vi "Periodic Tasks.vi"() -> ()   [LabVIEW 2011]
doc: "This VI runs in parallel to other tasks. It can contain as many user-defined periodic loops as you need. These can carry out PID or other sorts of timed response."
uses:
  <vilib>/Rock Robotics/SystemInterfaces/Utilities/FPGA_UtilitiesLED State.ctl
  <vilib>/Rock Robotics/SystemInterfaces/Utilities/FPGA_UtilitiesLED Source.ctl
  Robot Global Data.vi
  <vilib>/Rock Robotics/WPI/Relay/WPI_RelayValue.ctl
panel:
  in  "Reset Ball":bool
  in  "Home Speed":dbl=0.4
  out "Auton Recording":bool
  in  "Turn on Record":bool
  in  "Auton Array":dbl[][](array[numeric])
  out "Ramp ACT Pot":dbl
  out "Right Rate":dbl
  out "Right Direction":bool
  out "Right Distance":dbl
  out "Shooter Encoder Distance":dbl
  out "Shooter Direction":bool
  out "Shooter Encoder Rate":dbl
  out "Left Rate":dbl
  out "Gyro Rate":dbl
  out "Gyro Angle":dbl
  out "Left Direction":bool
  out "Left Distance":dbl
  # "Auton Recording"
  # "Sensor Feedback"
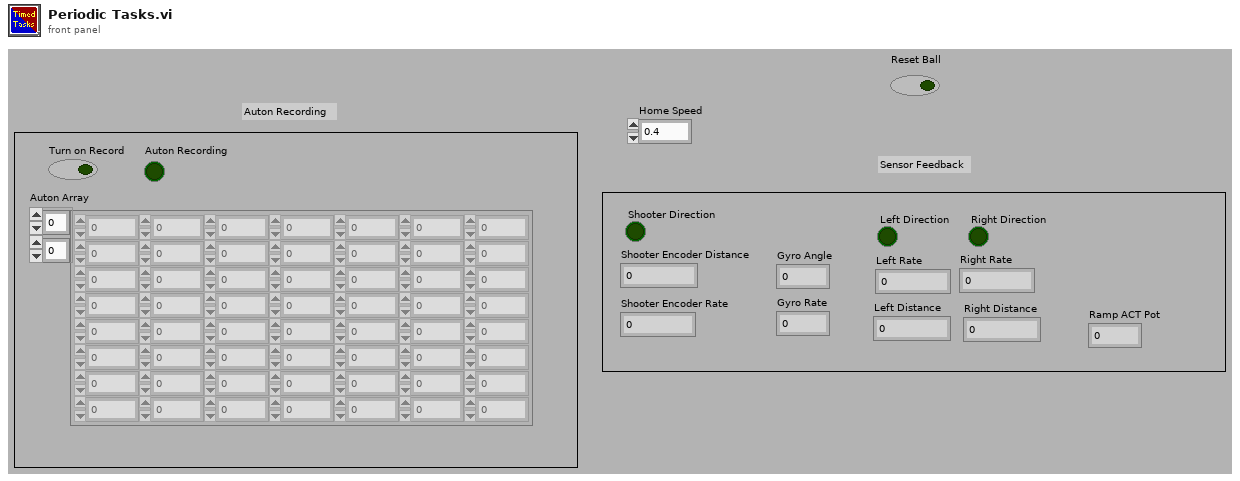
[diagram p1: front panel]
types:
  T1 = typedef "WPI_RelayValue.ctl" = enum16{"Off", "On", "Forward", "Reverse"}
  T2 = typedef "WPI_AnalogChannelDevRef.ctl" = cluster{"DevStatus":errorcluster, "Analog Module":T3, "Analog Channel":T4}
  T3 = typedef "FPGA_TypedefAnalogModule.ctl" = enum16{"Analog Module 1", "Analog Module 2"}
  T4 = typedef "FPGA_AIChannel.ctl" = enum8{"AI 1", "AI 2", "AI 3", "AI 4", "AI 5", "AI 6", "AI 7", "AI 8", "Invalid"}
  T5 = typedef "WPI_EncoderDevRef.ctl" = cluster{"DevStatus":errorcluster, "EncoderIndex":T6, "CounterIndex":T7, "DistancePerCount":dbl, "Decoding Type":T8}
  T6 = typedef "FPGA_EncoderIdx.ctl" = enum8{"Enc 0", "Enc 1", "Enc 2", "Enc 3", "Invalid"}
  T7 = typedef "FPGA_CounterCtrSystemIndex.ctl" = enum8{"Ctr 0", "Ctr 1", "Ctr 2", "Ctr 3", "Ctr 4", "Ctr 5", "Ctr 6", "Ctr 7", "Invalid"}
  T8 = typedef "WPI_EncoderType.ctl" = enum16{"1x", "2x", "4x"}
  T9 = typedef "WPI_GyroDevRef.ctl" = cluster{"DevStatus":errorcluster, "Analog Module":T3, "Analog Channel":T4, "Offset":dbl, "Gain (VoltsPerDegree/Second)":dbl}
  T10 = typedef "WPI_RelayDevRef.ctl" = cluster{"DevStatus":errorcluster, "Relay Channel":T11, "Digital Module":T12, "Relay Direction":T13}
  T11 = typedef "FPGA_DIORelayChannel.ctl" = enum8{"Relay 1", "Relay 2", "Relay 3", "Relay 4", "Relay 5", "Relay 6", "Relay 7", "Relay 8", "Invalid"}
  T12 = typedef "FPGA_TypedefDigitalModule.ctl" = enum16{"Digital Module 1", "Digital Module 2"}
  T13 = typedef "WPI_RelayDirection.ctl" = enum16{"Both directions", "Forward only", "Reverse only"}
  T14 = typedef "FPGA_UtilitiesLED State.ctl" = enum16{"Off", "On", "Toggle"}
  T15 = typedef "FPGA_UtilitiesLED Source.ctl" = enum16{"User LED", "FPGA LED"}
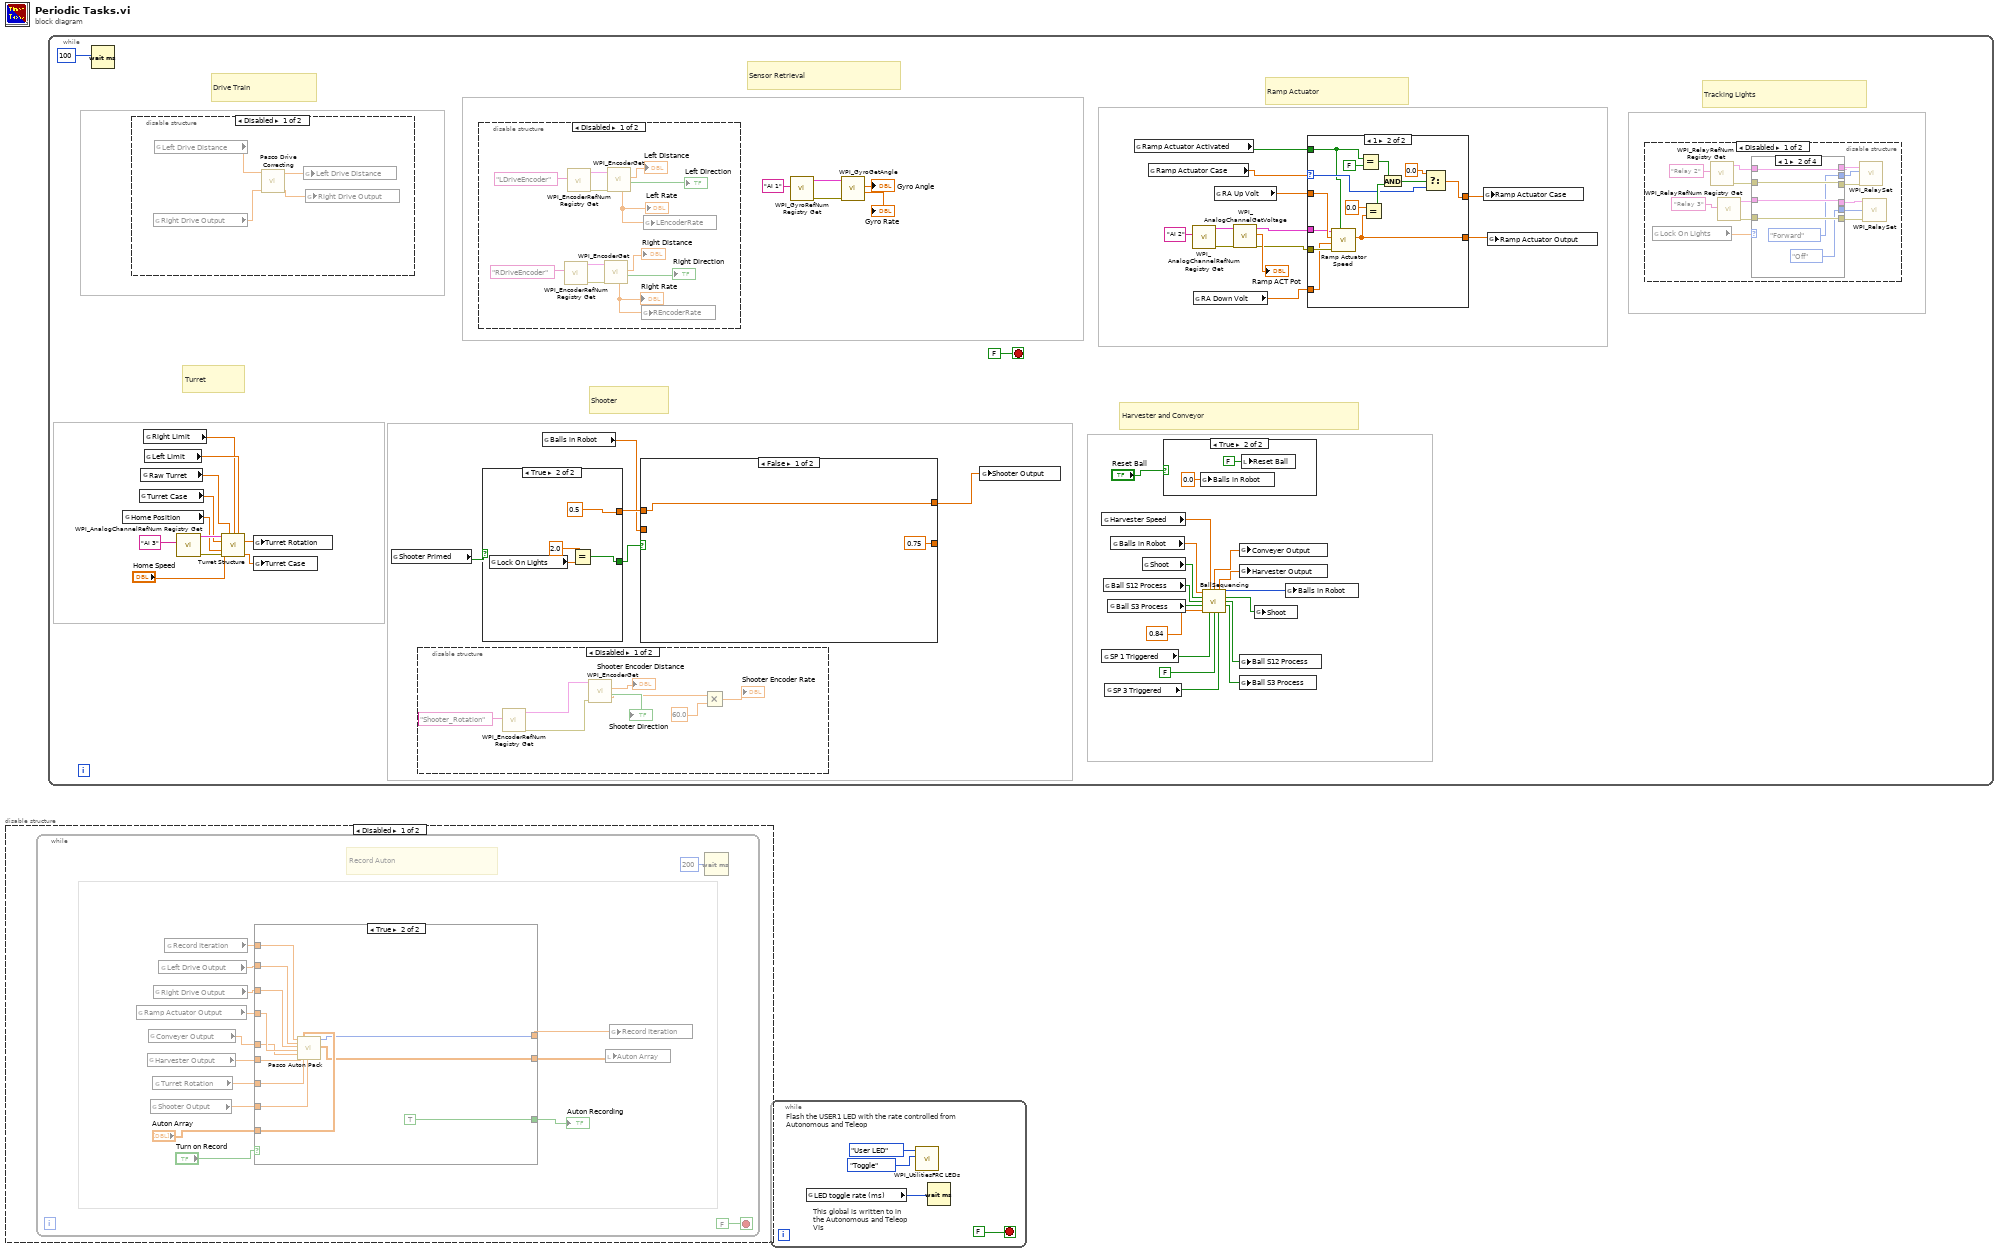
[diagram p0: block diagram]
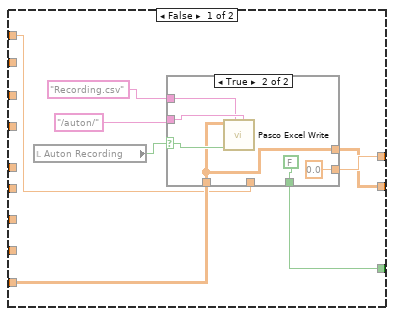
[diagram p2: hidden frame]
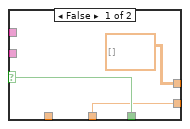
[diagram p3: hidden frame]
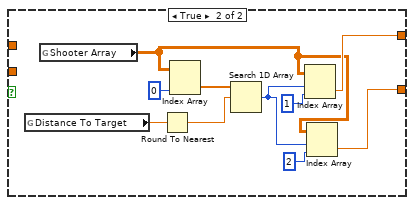
[diagram p5: hidden frame]
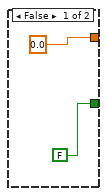
[diagram p6: hidden frame]
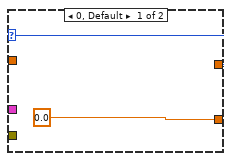
[diagram p8: hidden frame]
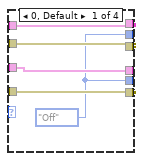
[diagram p10: hidden frame]
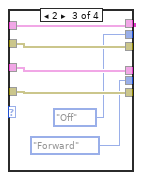
[diagram p11: hidden frame]
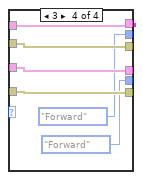
[diagram p12: hidden frame]
diagram:
  n1 = disable-structure shown="Disabled" {
    frame Disabled {
      n2 = while {
        stop <- FALSE stop-if-true
        # "Record Auton"
        n3 = global read "Robot Global Data.vi" "Ramp Actuator Output"() -> (w5:dbl)
        n4 = global read "Robot Global Data.vi" "Harvester Output"() -> (w7:dbl)
        n5 = global read "Robot Global Data.vi" "Conveyer Output"() -> (w6:dbl)
        n6 = global read "Robot Global Data.vi" "Shooter Output"() -> (w9:dbl)
        n7 = global read "Robot Global Data.vi" "Turret Rotation"() -> (w8:dbl)
        n8 = global read "Robot Global Data.vi" "Right Drive Output"() -> (w4:dbl)
        n9 = global read "Robot Global Data.vi" "Left Drive Output"() -> (w3:dbl)
        n10 = global read "Robot Global Data.vi" "Record Iteration"() -> (w2:dbl)
        n11 = case shown="True" "Turn on Record" {
          tunnel: w2 -> [w19 w44]
          tunnel: w3 -> [_ w43]
          tunnel: w4 -> [_ w42]
          tunnel: w5 -> [_ w41]
          tunnel: w6 -> [_ w40]
          tunnel: w7 -> [_ w39]
          tunnel: w8 -> [_ w38]
          tunnel: w9 -> [_ w37]
          tunnel: "Auton Array" -> [w20 w36]
          tunnel: [w16 w35] -> w12
          tunnel: [w17 w34] -> w13
          tunnel: [w18 TRUE] -> w14
          frame False {
            n12 = local read "Auton Recording"() -> (w21:bool)
            n13 = case shown="True" w21 {
              selector: w21 -> [w26 w31]
              tunnel: [w26 FALSE] -> w18
              tunnel: "/auton/" ("File Name") -> [_ w30]
              tunnel: "Recording.csv" ("Folder Location") -> [_ w29]
              tunnel: [w25 0.0 ("Record Iteration")] -> w17
              tunnel: w19 -> [w25 _]
              tunnel: w20 -> [_ w27]
              tunnel: [dbl[][] [] ("Auton Array") w27] -> w16
              frame False {
              }
              frame True {
                n14 = call "Pasco Excel Write.vi"("Folder Location"=w30, "File Name"=w29, "WriteToExcel"=w31, "2D data"=w27) -> ()  [unwired: 7 in, 1 out]
              }
            }
          }
          frame True {
            n15 = call "Pasco Auton Pack.vi"("Iterations"=w44, "Left Drive"=w43, "Right Drive"=w42, "RAMP ACT"=w41, "Conveyor"=w40, "Harvestor"=w39, "Auton Array"=w36, "Turret"=w38, "Shooter"=w37) -> ("Iteration Output"=w34:i32, "output array"=w35:dbl[][])  [unwired: 9 in]
          }
        }
        "Auton Recording" <- w14
        n16 = local write "Auton Array"(w12) -> ()
        n17 = global write "Robot Global Data.vi" "Record Iteration"(w13) -> ()
        n18 = Wait (ms)(milliseconds to wait=u32 200) -> ()  [unwired: 1 out]
      }
    }
    frame Enabled {
    }
  }
  n19 = while {
    stop <- FALSE stop-if-true
    # "Tracking Lights"
    # "Harvester and Conveyor"
    # "Shooter"
    # "Sensor Retrieval"
    # "Turret"
    # "Drive Train"
    # "Ramp Actuator"
    n20 = Wait (ms)(milliseconds to wait=u32 100) -> ()  [unwired: 1 out]
    n21 = global read "Robot Global Data.vi" "Home Position"() -> (w89:dbl)
    n22 = disable-structure shown="Disabled" {
      frame Disabled {
        n23 = global read "Robot Global Data.vi" "Right Drive Output"() -> (w182:dbl)
        n24 = global read "Robot Global Data.vi" "Left Drive Distance"() -> (w183:dbl)
        n25 = call "Pasco Drive Correcting.vi"("RightDriveOutput"=w182, "LeftDriveOutput"=w183) -> ("RightDriveOutput"=w180:dbl, "LeftDriveOutput"=w181:dbl)  [unwired: 8 in]
        n26 = global write "Robot Global Data.vi" "Left Drive Distance"(w181) -> ()
        n27 = global write "Robot Global Data.vi" "Right Drive Output"(w180) -> ()
      }
      frame Enabled {
      }
    }
    n28 = global read "Robot Global Data.vi" "Turret Case"() -> (w90:dbl)
    n29 = global read "Robot Global Data.vi" "Raw Turret"() -> (w88:dbl)
    n30 = global read "Robot Global Data.vi" "Right Limit"() -> (w71:dbl)
    n31 = global read "Robot Global Data.vi" "Left Limit"() -> (w72:dbl)
    n32 = call <vilib>:"WPI_AnalogChannelRefNum Registry Get.vi"("refnum name"="AI 3") -> ("error out"=w91:errorcluster, "AIDeviceRef"=w92:T2)  [unwired: 9 in]
    n33 = call "Turret Structure.vi"("AIDeviceRef"=w92, "Raw Turret"=w88, "upper limit"=w71, "lower limit"=w72, "Turret Case"=w90, "Home Speed"="Home Speed", "Home postion"=w89, "error in (no error)"=w91) -> ("Turret Output"=w87:dbl, "Turret Case Output"=w86:dbl)  [unwired: 6 in]
    n34 = global write "Robot Global Data.vi" "Turret Rotation"(w87) -> ()
    n35 = global write "Robot Global Data.vi" "Turret Case"(w86) -> ()
    n36 = global read "Robot Global Data.vi" "Shooter Primed"() -> (w58:bool)
    n37 = disable-structure shown="Disabled" {
      frame Disabled {
        n38 = call <vilib>:"WPI_EncoderRefNum Registry Get.vi"("refnum name"="Shooter_Rotation") -> ("error out"=w184:errorcluster, "EncoderDevRef"=w185:T5)  [unwired: 9 in]
        n39 = call <vilib>:"WPI_EncoderGet.vi"("error in (no error)"=w184, "EncoderDevRef"=w185) -> ("Direction"=→"Shooter Direction":bool, "Distance"=→"Shooter Encoder Distance":dbl, "Rate"=w188:dbl)  [unwired: 4 in, 3 out]
        n40 = Multiply(x=w188, y=60.0) -> (x*y=→"Shooter Encoder Rate":dbl)
      }
      frame Enabled {
      }
    }
    n41 = disable-structure shown="Disabled" {
      frame Disabled {
        n42 = call <vilib>:"WPI_EncoderRefNum Registry Get.vi"("refnum name"="RDriveEncoder") -> ("error out"=w136:errorcluster, "EncoderDevRef"=w135:T5)  [unwired: 9 in]
        n43 = call <vilib>:"WPI_EncoderRefNum Registry Get.vi"("refnum name"="LDriveEncoder") -> ("error out"=w142:errorcluster, "EncoderDevRef"=w141:T5)  [unwired: 9 in]
        n44 = call <vilib>:"WPI_EncoderGet.vi"("error in (no error)"=w136, "EncoderDevRef"=w135) -> ("Direction"=→"Right Direction":bool, "Distance"=→"Right Distance":dbl, "Rate"=w132:dbl)  [unwired: 4 in, 3 out]
        "Right Rate" <- w132
        n45 = call <vilib>:"WPI_EncoderGet.vi"("error in (no error)"=w142, "EncoderDevRef"=w141) -> ("Direction"=→"Left Direction":bool, "Distance"=→"Left Distance":dbl, "Rate"=w138:dbl)  [unwired: 4 in, 3 out]
        "Left Rate" <- w138
        n46 = global write "Robot Global Data.vi" "REncoderRate"(w132) -> ()
        n47 = global write "Robot Global Data.vi" "LEncoderRate"(w138) -> ()
      }
      frame Enabled {
      }
    }
    n48 = case shown="True" w58 {
      tunnel: [FALSE ("Shooter Primed") w110] -> w57
      tunnel: [0.0 0.5] -> w55
      frame False {
      }
      frame True {
        n49 = global read "Robot Global Data.vi" "Lock On Lights"() -> (w112:dbl)
        n50 = Equal?(x=2.0, y=w112) -> (x = y?=w110:bool)
      }
    }
    n51 = global read "Robot Global Data.vi" "Balls in Robot"() -> (w54:dbl)
    n52 = case shown="False" w57 {
      tunnel: [w97 w107] -> w56
      tunnel: w55 -> [w97 _]
      tunnel: w54 -> [_ _]
      tunnel: [0.75 w106] -> _
      frame False {
      }
      frame True {
        n53 = global read "Robot Global Data.vi" "Distance To Target"() -> (w103:dbl)
        n54 = global read "Robot Global Data.vi" "Shooter Array"() -> (w98:dbl[][])
        n55 = Round To Nearest(number=w103) -> (nearest integer value=w102:dbl)
        n56 = Index Array(array=w98, index (col)=0 ("disabled index (col)")) -> (element=w101:dbl[])  [unwired: 1 in]
        n57 = Search 1D Array(1D array=w101, element=w102) -> (index of element=w99:i32)  [unwired: 1 in]
        n58 = Index Array(array=w98, index (row)=w99, index (col)=1 ("disabled index (col)")) -> (element=w107:dbl)
        n59 = Index Array(array=w98, index (row)=w99, index (col)=2 ("disabled index (col)")) -> (element=w106:dbl)
      }
    }
    n60 = call <vilib>:"WPI_GyroRefNum Registry Get.vi"("refnum name"="AI 1") -> ("error out"=w51:errorcluster, "GyroDevRef"=w52:T9)  [unwired: 9 in]
    n61 = call <vilib>:"WPI_GyroGetAngle.vi"("error in (no error)"=w51, "GyroDevRef"=w52) -> ("Angular Rate"=→"Gyro Rate":dbl, "Angle"=→"Gyro Angle":dbl)  [unwired: 6 in, 2 out]
    n62 = global write "Robot Global Data.vi" "Shooter Output"(w56) -> ()
    n63 = global read "Robot Global Data.vi" "Harvester Speed"() -> (w53:dbl)
    n64 = global read "Robot Global Data.vi" "SP 1 Triggered"() -> (w62:bool)
    n65 = global read "Robot Global Data.vi" "Ball S12 Process"() -> (w64:bool)
    n66 = global read "Robot Global Data.vi" "SP 3 Triggered"() -> (w61:bool)
    n67 = global read "Robot Global Data.vi" "Ball S3 Process"() -> (w63:bool)
    n68 = global read "Robot Global Data.vi" "Balls in Robot"() -> (w66:dbl)
    n69 = global read "Robot Global Data.vi" "Ramp Actuator Activated"() -> (w79:bool)
    n70 = global read "Robot Global Data.vi" "Shoot"() -> (w65:bool)
    n71 = global read "Robot Global Data.vi" "Ramp Actuator Case"() -> (w81:dbl)
    n72 = case shown="True" "Reset Ball" {
      frame False {
      }
      frame True {
        n73 = global write "Robot Global Data.vi" "Balls in Robot"(0.0 ("Balls in Robot")) -> ()
        n74 = local write "Reset Ball"(FALSE ("Reset Ball")) -> ()
      }
    }
    n75 = call <vilib>:"WPI_AnalogChannelRefNum Registry Get.vi"("refnum name"="AI 2") -> ("error out"=w77:errorcluster, "AIDeviceRef"=w78:T2)  [unwired: 9 in]
    n76 = global read "Robot Global Data.vi" "RA Down Volt"() -> (w84:dbl)
    n77 = call "BallSequencing.vi"("Balls In Robot"=w66, "Speed of Harvester"=w53, "Shoot"=w65, "Ball S12 Process"=w64, "Ball S3 Process"=w63, "Speed of Conveyor"=0.84, "SP 1 Triggered"=w62, "SP 2 Triggered"=FALSE, "SP 3 Triggered"=w61) -> ("Conveyer Output"=w67:dbl, "Harvester Output"=w68:dbl, "Balls In Robot Output"=w46:i32, "Shoot Output"=w45:bool, "Ball S12 Process Output"=w70:bool, "Ball S3 Process Output"=w69:bool)  [unwired: 1 in]
    n78 = global read "Robot Global Data.vi" "RA Up Volt"() -> (w83:dbl)
    n79 = call <vilib>:"WPI_AnalogChannelGetVoltage.vi"("error in (no error)"=w77, "AIDeviceRef"=w78) -> ("error out"=w74:errorcluster, "Voltage"=→"Ramp ACT Pot":dbl, "AIDeviceRef"=w75:T2)  [unwired: 7 in]
    n80 = global write "Robot Global Data.vi" "Conveyer Output"(w67) -> ()
    n81 = global write "Robot Global Data.vi" "Harvester Output"(w68) -> ()
    n82 = global write "Robot Global Data.vi" "Ball S12 Process"(w70) -> ()
    n83 = global write "Robot Global Data.vi" "Ball S3 Process"(w69) -> ()
    n84 = global write "Robot Global Data.vi" "Shoot"(w45) -> ()
    n85 = global write "Robot Global Data.vi" "Balls in Robot"(w46) -> ()
    n86 = case shown="1" w81 {
      selector: w81 -> [w116 w121]
      tunnel: w74 -> [_ w131]
      tunnel: w84 -> [_ w130]
      tunnel: w83 -> [_ w129]
      tunnel: [0.0 ("Ramp Actuator Ouput") w120] -> w82
      tunnel: w79 -> [_ w119]
      tunnel: [w116 w122] -> w80
      tunnel: w75 -> [_ w118]
      frame 0, Default {
      }
      frame 1 {
        n87 = call "Ramp Actuator Speed.vi"("Up to Down"=w119, "error in (no error)"=w131, "RA Down Volt"=w130, "RA Up Volt"=w129, "AIDeviceRef"=w118) -> ("Ramp Actuator Ouput"=w120:dbl)  [unwired: 6 in]
        n88 = Equal?(x=w119, y=FALSE) -> (x = y?=w126:bool)
        n89 = Equal?(x=0.0, y=w120) -> (x = y?=w127:bool)
        n90 = And(x=w126, y=w127) -> (x .and. y?=w124:bool)
        n91 = Select(t=0.0, s=w124, f=w121) -> (s? t:f=w122:dbl)
      }
    }
    n92 = global write "Robot Global Data.vi" "Ramp Actuator Case"(w80) -> ()
    n93 = global write "Robot Global Data.vi" "Ramp Actuator Output"(w82) -> ()
    n94 = disable-structure shown="Disabled" {
      frame Disabled {
        n95 = global read "Robot Global Data.vi" "Lock On Lights"() -> (w144:dbl)
        n96 = call <vilib>:"WPI_RelayRefNum Registry Get.vi"("refnum name"="Relay 2") -> ("error out"=w151:errorcluster, "RelayDevRef"=w153:T10)  [unwired: 9 in]
        n97 = call <vilib>:"WPI_RelayRefNum Registry Get.vi"("refnum name"="Relay 3") -> ("error out"=w148:errorcluster, "RelayDevRef"=w149:T10)  [unwired: 9 in]
        n98 = case shown="1" w144 {
          tunnel: [w161 w167 w173 w179] -> w154
          tunnel: w153 -> [w161 w167 w173 w179]
          tunnel: [w160 w166 w172 w178] -> w152
          tunnel: w151 -> [w160 w166 w172 w178]
          tunnel: [w159 w165 w171 w177] -> w150
          tunnel: w149 -> [w159 w165 w171 w177]
          tunnel: w148 -> [w158 w164 w170 w176]
          tunnel: [w158 w164 w170 w176] -> w147
          tunnel: [w157 WPI_RelayValue."Forward" ("RelayValue") WPI_RelayValue."Off" ("RelayValue") WPI_RelayValue."Forward" ("RelayValue")] -> w146
          tunnel: [w157 WPI_RelayValue."Off" ("RelayValue") WPI_RelayValue."Forward" ("RelayValue") WPI_RelayValue."Forward" ("RelayValue")] -> w145
          frame 0, Default {
            w157 = WPI_RelayValue."Off" ("RelayValue")
          }
          frame 1 {
          }
          frame 2 {
          }
          frame 3 {
          }
        }
        n99 = call <vilib>:"WPI_RelaySet.vi"("error in (no error)"=w152, "RelayValue"=w146, "RelayDevRef"=w154) -> ()  [unwired: 7 in, 2 out]
        n100 = call <vilib>:"WPI_RelaySet.vi"("error in (no error)"=w147, "RelayValue"=w145, "RelayDevRef"=w150) -> ()  [unwired: 7 in, 2 out]
      }
      frame Enabled {
      }
    }
  }
  n101 = while {
    stop <- FALSE stop-if-true
    # "This global is written to in the Autonomous and Teleop VIs"
    # "Flash the USER1 LED with the rate controlled from Autonomous and Teleop"
    n102 = global read "Robot Global Data.vi" "LED toggle rate (ms)"() -> (w192:u32)
    n103 = call <vilib>:"WPI_UtilitiesFRC LEDs.vi"("State"=FPGA_UtilitiesLED_State."Toggle", "LED Type"=FPGA_UtilitiesLED_Source."User LED") -> ()  [unwired: 1 in, 9 out]
    n104 = Wait (ms)(milliseconds to wait=w192) -> ()  [unwired: 1 out]
  }
